vi "decimate_waveforms.vi"(8 "error in (no error)":errorcluster, 10 "WFM":waveform(dbl)[](array[waveform]), 11 "LockinDAQ":refnum<class "Lockin.DAQ.lvclass">) -> (0 "error out":errorcluster, 2 "WFM out":waveform(dbl)[](array[waveform]), 3 "LockinDAQ out":refnum<class "Lockin.DAQ.lvclass">)   [LabVIEW 2016, in "Lockin.DAQ.lvclass"]
doc: "Decimates the input sequence X by the decimating factor and the averaging Boolean control."
uses:
  Lockin.DAQ.lvclass
  Lockin.DAQ.lvclass/Lockin.DAQ.ctl
  <vilib>/Analysis/2dsp.llb/Decimate (single shot, DBL).vi
  <vilib>/Analysis/NI_AALPro.lvlib
  <vilib>/addons/Digital Filter Design/NI_DigFilterLicensed.lvlib
  <vilib>/addons/Digital Filter Design/Design.llb/DFD MRate Filter Design (Integer).vi
  <vilib>/addons/Digital Filter Design/Multirate.llb/DFD MRate Filtering with State (Wfm).vi
panel:
  # "by Marco Tedaldi, Brain Research Institute, University of Zurich, 2013"
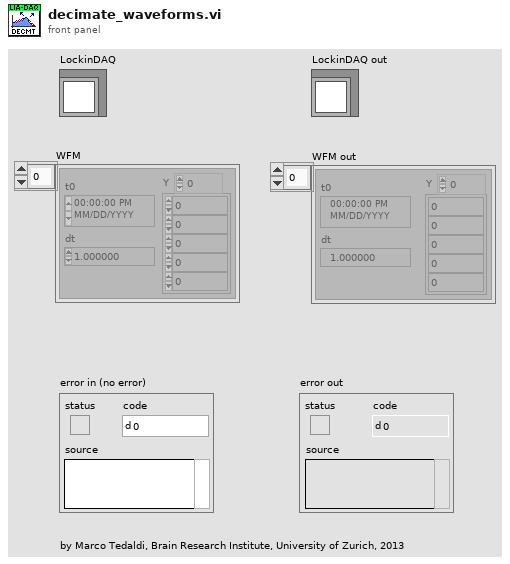
[diagram p1: front panel]
types:
  T1 = typedef "NI_DigFilterLicensed.lvlib/DFD Multirate Filter Obj.ctl" = cluster{"mMRate_Structure":enum16{"CIC", "FIR", "IIR", "Lattice"}, "mMRate_Mode":T2, "mMRate_Factor":i32, "mMRate_FIRParams":cluster{"mMRate_FIR_H":dbl[], "mMRate_FIR_IsNyquist?":bool, "mMRate_FIR_IsSymmetric?":bool}, "mMRate_CICParams":cluster{"mMRate_CIC_#Stage":i32, "mMRate_CIC_Lag":i32, "mMRate_CIC_Type":enum16{"Lowpass", "Highpass"}}, "mMRate_Order":i32, "mMRate_Version":string, "mMRate_Comments":string, "mMRate_RationalFactor":cluster{"mMRate_L":i32, "mMRate_M":i32}, "mMRate_Fs":dbl, "mMRate_Quantized?":bool, "mMRate_QFilterGain":dbl, "mMRate_CoefWl":i16, "mMRate_Scaling":cluster{"mMRate_ScaleByPowerOf2?":bool, "mMRate_ScaleType":T3}, "mMRate_InputWl":i16, "mMRate_OutputWl":i16, "mMRate_OutputMode":T4, "mMRate_MultMode":T5, "mMRate_BitPruning":bool, "mMRate_GainWl":i16, "mMRate_OutputFwl":i16, "mMRate_SumIwl":i16, "mMRate_InputIwl ":i16, "mMRate_SumWl":i16, "mMRate_CoefIwl":i16}
  T2 = typedef "NI_DigFilterLicensed.lvlib/DFD Multirate Mode.ctl" = i16
  T3 = typedef "NI_DigFilterLicensed.lvlib/DFD Coef Norm Type.ctl" = enum16{"No Norm", "Time Domain 1-Norm", "Time Domain 2-Norm", "Time Domain Inf-Norm"}
  T4 = typedef "NI_DigFilterLicensed.lvlib/DFD Round-off Mode.ctl" = enum16{"Nearest", "Truncation"}
  T5 = typedef "NI_DigFilterLicensed.lvlib/DFD FXP MRate Multiply Mode.ctl" = enum16{"Truncated", "Full"}
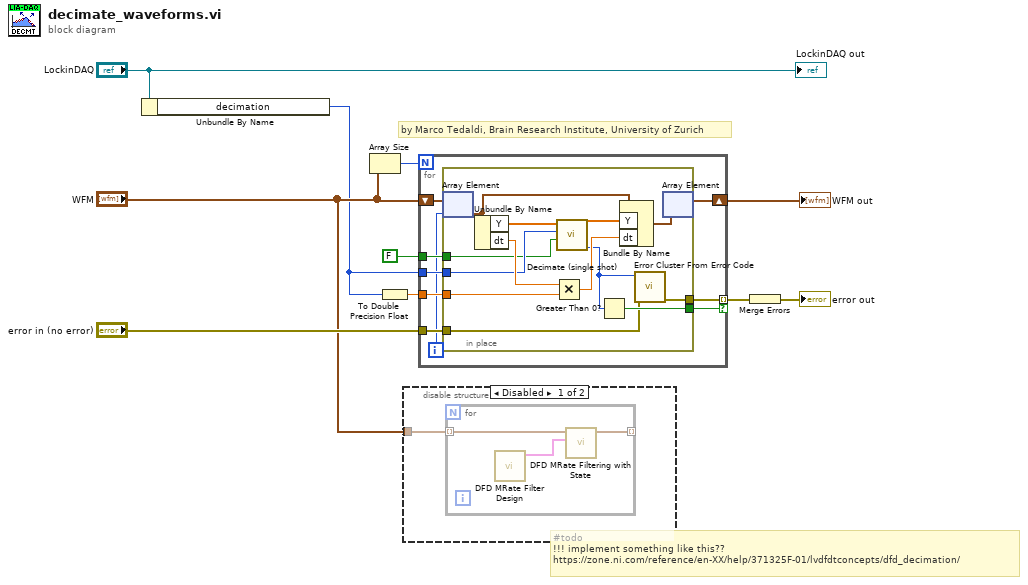
[diagram p0: block diagram]
diagram:
  # "#todo\n!!! implement something like this??\nhttps://zone.ni.com/reference/en-XX/help/371325F-01/lvdfdtconcepts/dfd_decimation/"
  # "by Marco Tedaldi, Brain Research Institute, University of Zurich"
  n1 = Unbundle By Name("LockinDAQ") -> ("decimation"=w1:u32)
  n2 = Array Size(array="WFM") -> (size(s)=w7:i32)
  n3 = To Double Precision Float(number=w1) -> (double precision float=w10:dbl)
  n4 = disable-structure shown="Disabled" {
    disable-tunnel: "WFM" -> [w11 _]
    frame Disabled {
      n5 = for {
        tunnel: w11 -> [w14] mode=indexing
        tunnel: [w13] -> _ mode=indexing
        n6 = call-poly <vilib>:"DFD MRate Filter Design.vi"() -> ("multirate filter out"=w12:T1)  [unwired: 10 in, 1 out]
        n7 = call-poly <vilib>:"DFD MRate Filtering with State.vi"("multirate filter"=w12, "signal in"=w14) -> ("signal out"=w13:waveform(dbl))  [unwired: 7 in, 2 out]
      }
    }
    frame Enabled {
    }
  }
  n8 = for {
    N: w7 -> [_]
    tunnel: w10 -> [w23]
    tunnel: w1 -> [w22]
    tunnel: FALSE ("averaging") -> [w21]
    tunnel: "error in (no error)" -> [w19]
    tunnel: [w18] -> w5 mode=indexing if=w20
    shift-right: [w15] -> w6
    shift-left: "WFM" -> [w17]
    i -> [w16]
    n9 = in-place {
      in-place-border: w23 -> [w33]
      in-place-border: w22 -> [w32]
      in-place-border: w21 -> [w30]
      in-place-border: [w29] -> w20
      in-place-border: w19 -> [w28]
      in-place-border: [w27] -> w18
      n10 = in-place-array #1(w17, w16) -> (w24:waveform(dbl))
      n11 = Unbundle By Name(w24) -> ("Y"=w36:dbl[], "dt"=w34:dbl)
      n12 = Multiply(x=w34, y=w33) -> (x*y=w31:dbl)
      n13 = call-poly <vilib>:"Decimate (single shot).vi"("averaging"=w30, "decimating factor"=w32, "X"=w36) -> ("error"=w26:i32, "Decimated Array"=w35:dbl[])  [unwired: 7 in]
      n14 = Greater Than 0?(x=w26) -> (x > 0?=w29:bool)
      n15 = Bundle By Name(cluster=w24, "Y"=w35, "dt"=w31) -> (w25:waveform(dbl))
      n16 = call <vilib>:"Error Cluster From Error Code.vi"("error in (no error)"=w28, "error code (0)"=w26) -> ("error out"=w27:errorcluster)  [unwired: 7 in]
      n17 = in-place-array #1(w25) -> (w15:waveform(dbl)[])  [unwired: 1 out]
    }
  }
  "WFM out" <- w6
  n18 = Merge Errors(w5) -> (→"error out":errorcluster)
  "LockinDAQ out" <- "LockinDAQ"
